vi "三角形.vi"() -> ()   [LabVIEW 2012]
panel:
  in  "y":dbl[](array[numeric])
  in  "x":dbl[](array[numeric])
  out "XY图":cluster{"x":dbl[], "y":dbl[]}(graph)
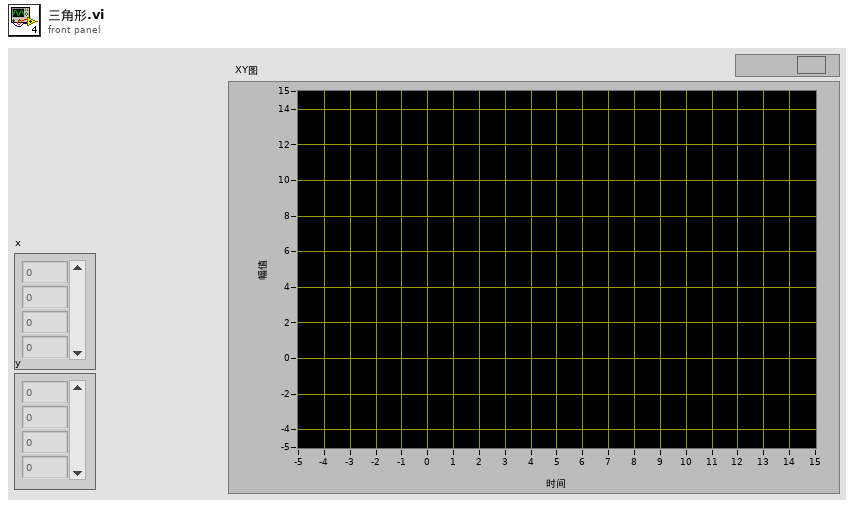
[diagram p1: front panel]
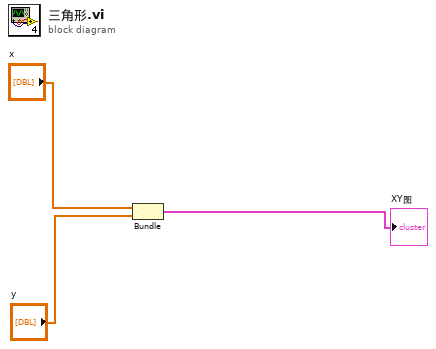
[diagram p0: block diagram]
diagram:
  n1 = Bundle("x"="x", "y"="y") -> (→"XY图":cluster{"x":dbl[], "y":dbl[]})  [unwired: 1 in]
